vi "Lab Panel V6.00.vi"() -> ()   [LabVIEW 2017] (continued)
                                n860 = local read "SET LAB03-2"() -> (w1506:T5)
                                n861 = case shown="\"T-RISE TEST\"" w1511 {
                                tunnel: ["L03-2-CHART TEST-" "L03-2-CYCLE TEST-" "L03-2-T-RISE TEST-"] -> w1507
                                frame "CHART TEST", Default {
                                }
                                frame "CYCLE TEST" {
                                }
                                frame "T-RISE TEST" {
                                }
                                }
                                n862 = Unbundle(w1506) -> ("DESCRIPTION"=w1505:string)  [unwired: 4 out]
                                n863 = Concatenate Strings(w1501, "\\", w1499, w1497, w1498, w1497) -> (w1508:string)
                                n864 = String To Path(string=w1508) -> (path=w1510:path)
                                n865 = Concatenate Strings(w1508, w1507, w1505, "-", w1504, ".tdms") -> (w1496:string)
                                n866 = Create Folder(path (use dialog)=w1510) -> (error out=w1509:errorcluster)  [unwired: 2 in, 2 out]
                                n867 = global write "Global 1.vi" "LAB03-2 FILE"(w1496) -> ()
                                n868 = call <vilib>:"Clear Errors.vi"("error in (no error)"=w1509) -> ()  [unwired: 5 in, 2 out]
                              }
                              frame #1 {
                                (unwired) FALSE
                                n869 = String To Path(string=w1520) -> (path=w1516:path)
                                n870 = TDMS Open(6:FALSE, 10:T22."create or replace" ("operation (0:open)"), 11:w1516) -> (0:w1515:errorcluster, 3:→"TDMS LAB03-2":refnum<k34>)  [unwired: 4 in]
                              }
                              frame #2 {
                                n871 = local read "SET LAB03-2"() -> (w1526:T5)
                                n872 = local read "TDMS LAB03-2"() -> (w1537:refnum<k34>)
                                n873 = Build Array("Testers Name", "Description", "Set Test Cycles", "T-Rise minutes", "T-Rise Deg C") -> (w1527:string[])
                                n874 = Unbundle(w1526) -> ("NAME"=w1525:string, "DESCRIPTION"=w1524:string, "CYCLES"=w1523:dbl, "T-RISE mins"=w1522:dbl, "T-RISE deg C"=w1521:dbl)
                                n875 = Number To Decimal String(number=w1523) -> (decimal integer string=w1536:string)  [unwired: 1 in]
                                n876 = Number To Decimal String(number=w1522) -> (decimal integer string=w1535:string)  [unwired: 1 in]
                                n877 = Number To Decimal String(number=w1521) -> (decimal integer string=w1534:string)  [unwired: 1 in]
                                n878 = Build Array(w1525, w1524, w1536, w1535, w1534) -> (w1533:string[])
                                n879 = TDMS Set Properties(5:w1533, 7:w1527, 11:w1537) -> ()  [unwired: 3 in, 4 out]
                              }
                              frame #3 {
                                n880 = local read "DISP LAB03-2"() -> (w1542:T4)
                                n881 = Concatenate Strings("LAB03-2  ", w1541) -> (w1543:string)
                                n882 = Two Button Dialog(message=w1543, 1:w1539, 2:w1540) -> (T button?=w1545:bool)
                                n883 = case shown="True" w1545 {
                                tunnel: w1542 -> [w1552 w1553]
                                tunnel: [w1552 w1553] -> w1549
                                tunnel: [w1551 w1554] -> w1548
                                tunnel: [w1550 w1554] -> w1547
                                frame False {
                                n884 = Unbundle(w1552) -> ("CYCLE"=w1551:dbl, "MINS"=w1550:dbl)  [unwired: 1 out]
                                }
                                frame True {
                                w1554 = 0.0
                                }
                                }
                                n885 = Bundle(cluster=w1549, "CYCLE"=w1548, "MINS"=w1547, "STATUS"="RUN") -> (w1538:T4)
                                n886 = local write "DISP LAB03-2"(w1538) -> ()
                              }
                              frame #4 {
                                n887 = local read "TEMP START LAB03-2"() -> (w1557:cluster{"TL":dbl, "TN":dbl})
                                n888 = Bundle(cluster=w1557, "TL"=w1555, "TN"=w1555) -> (w1556:cluster{"TL":dbl, "TN":dbl})
                                n889 = local write "TEMP START LAB03-2"(w1556) -> ()
                              }
                            }
                          }
                        }
                      }
                    }
                  }
                }
              }
              event "RUN LAB04-1": Value Change {
                n890 = event-data() -> ("NewVal"=w1562:bool)  [unwired: 1 in, 5 out]
                n891 = local write "run lab04-1"(w1562) -> ()
                n892 = case shown="True" w1562 {
                  tunnel: w1568 -> [_ w1606]
                  tunnel: w1567 -> [_ w1605]
                  tunnel: w1565 -> [w1570 w1604]
                  tunnel: w1566 -> [_ w1603]
                  tunnel: w1564 -> [_ w1602]
                  tunnel: [w1569 w1601] -> w1563
                  tunnel: w1561 -> [_ w1600]
                  tunnel: w1560 -> [_ w1599]
                  tunnel: w1559 -> [_ w1598]
                  tunnel: w1558 -> [_ w1596]
                  frame False {
                    # "stop test"
                    n893 = stacked-sequence {
                      tunnel: w1570 -> [w1579 _]
                      tunnel: [w1571 _] -> w1569
                      frame #0 {
                        n894 = local read "DISP LAB04-1"() -> (w1578:T4)
                        n895 = Unbundle(w1578) -> ("CYCLE"=w1576:dbl, "MINS"=w1577:dbl)  [unwired: 1 out]
                        n896 = case shown="\"CYCLE TEST\"" w1579 {
                          tunnel: w1577 -> [_ _ w1586]
                          tunnel: w1576 -> [w1584 w1585 _]
                          tunnel: [w1584 w1585 w1586] -> w1575
                          frame "CHART TEST", Default {
                          }
                          frame "CYCLE TEST" {
                          }
                          frame "T-RISE TEST" {
                          }
                        }
                        n897 = local read "TDMS LAB04-1"() -> (w1583:refnum<k34>)
                        n898 = Build Array("STOPPED") -> (w1580:string[])
                        n899 = Build Array(w1575) -> (w1574:dbl[])
                        n900 = TDMS Write(0:w1583, 5:"TEST RESULT", 7:w1580, 9:w1574) -> (4:w1572:refnum<k34>, 15:w1573:errorcluster)  [unwired: 2 in, 2 out]
                        n901 = TDMS Close(8:w1573, 11:w1572) -> (0:w1571:errorcluster)  [unwired: 1 out]
                      }
                      frame #1 {
                        n902 = local read "DISP LAB04-1"() -> (w1590:T4)
                        n903 = stacked-sequence {
                          tunnel: "LAB04-1" -> [w1592 w1594]
                          frame #0 {
                            n904 = call "sub vi - defrag tdms v1.vi"("panel id"=w1592) -> ("error out"=w1591:errorcluster)  [unwired: 10 in]
                            n905 = local write "data file error"(w1591) -> ()
                          }
                          frame #1 {
                            n906 = call "Save data file (stop) v3.vi"("panel id"=w1594) -> ("network file save error"=w1593:errorcluster)  [unwired: 9 in, 1 out]
                            n907 = local write "RESULT LAB04-1"(FALSE) -> ()
                            n908 = local write "data file error"(w1593) -> ()
                          }
                        }
                        n909 = Bundle(cluster=w1590, "STATUS"="STOP") -> (w1588:T4)  [unwired: 2 in]
                        n910 = local write "DISP LAB04-1"(w1588) -> ()
                      }
                    }
                  }
                  frame True {
                    n911 = local read "SIG LAB04-1"() -> (w1597:T2)
                    n912 = stacked-sequence {
                      seq-local: [w1608 _] -> [_ w1612]
                      tunnel: w1606 -> [_ w1622]
                      tunnel: w1605 -> [_ w1621]
                      tunnel: w1604 -> [_ w1620]
                      tunnel: w1603 -> [_ w1619]
                      tunnel: w1602 -> [_ w1618]
                      tunnel: [_ w1617] -> w1601
                      tunnel: w1600 -> [_ w1616]
                      tunnel: w1599 -> [_ w1615]
                      tunnel: w1598 -> [_ w1614]
                      tunnel: w1597 -> [w1607 w1613]
                      tunnel: w1596 -> [_ w1611]
                      frame #0 {
                        n913 = Unbundle(w1607) -> ("AMPS"=w1610:dbl)  [unwired: 4 out]
                        n914 = call "Check For Amps on v1.vi"("ID"="LAB04-1", "amps"=w1610) -> ("amps"=w1608:bool)  [unwired: 9 in]
                      }
                      frame #1 {
                        n915 = case shown="True" w1612 {
                          tunnel: w1622 -> [_ w1635]
                          tunnel: w1621 -> [_ w1634]
                          tunnel: w1620 -> [_ w1633]
                          tunnel: w1619 -> [_ w1632]
                          tunnel: w1618 -> [_ w1631]
                          tunnel: [errorcluster {"status"=FALSE, "code"=0, "source"=""} ("error out") w1630] -> w1617
                          tunnel: w1616 -> [_ w1629]
                          tunnel: w1615 -> [_ w1628]
                          tunnel: w1614 -> [_ w1627]
                          tunnel: w1613 -> [_ w1626]
                          tunnel: w1611 -> [_ w1625]
                          frame False {
                            w1623 = FALSE
                            n916 = local write "RUN LAB04-1"(w1623) -> ()
                            n917 = local write "run lab04-1"(w1623) -> ()
                          }
                          frame True {
                            n918 = stacked-sequence {
                              seq-local: [w1636 _ _ _ _] -> [_ w1660 _ _ _]
                              tunnel: w1635 -> [w1641 _ _ _ _]
                              tunnel: w1634 -> [w1637 _ _ _ _]
                              tunnel: w1633 -> [w1651 _ _ _ _]
                              tunnel: w1632 -> [w1644 _ _ _ _]
                              tunnel: w1631 -> [w1639 _ _ _ _]
                              tunnel: [_ w1655 _ _ _] -> w1630
                              tunnel: w1629 -> [_ _ _ w1681 _]
                              tunnel: w1628 -> [_ _ _ w1680 _]
                              tunnel: w1627 -> [_ _ _ w1679 _]
                              tunnel: w1626 -> [_ _ _ _ _]
                              tunnel: w1625 -> [_ _ _ _ w1695]
                              frame #0 {
                                w1638 = "\\"
                                n919 = local read "SET LAB04-1"() -> (w1646:T5)
                                n920 = case shown="\"CYCLE TEST\"" w1651 {
                                tunnel: ["L04-1-CHART TEST-" "L04-1-CYCLE TEST-" "L04-1-T-RISE TEST-"] -> w1647
                                frame "CHART TEST", Default {
                                }
                                frame "CYCLE TEST" {
                                }
                                frame "T-RISE TEST" {
                                }
                                }
                                n921 = Unbundle(w1646) -> ("DESCRIPTION"=w1645:string)  [unwired: 4 out]
                                n922 = Concatenate Strings(w1641, "\\", w1639, w1638, w1637, w1638) -> (w1648:string)
                                n923 = String To Path(string=w1648) -> (path=w1650:path)
                                n924 = Concatenate Strings(w1648, w1647, w1645, "-", w1644, ".tdms") -> (w1636:string)
                                n925 = Create Folder(path (use dialog)=w1650) -> (error out=w1649:errorcluster)  [unwired: 2 in, 2 out]
                                n926 = global write "Global 1.vi" "LAB04-1 FILE"(w1636) -> ()
                                n927 = call <vilib>:"Clear Errors.vi"("error in (no error)"=w1649) -> ()  [unwired: 5 in, 2 out]
                              }
                              frame #1 {
                                (unwired) FALSE
                                n928 = String To Path(string=w1660) -> (path=w1656:path)
                                n929 = TDMS Open(6:FALSE, 10:T22."create or replace" ("operation (0:open)"), 11:w1656) -> (0:w1655:errorcluster, 3:→"TDMS LAB04-1":refnum<k34>)  [unwired: 4 in]
                              }
                              frame #2 {
                                n930 = local read "SET LAB04-1"() -> (w1666:T5)
                                n931 = local read "TDMS LAB04-1"() -> (w1677:refnum<k34>)
                                n932 = Build Array("Testers Name", "Description", "Set Test Cycles", "T-Rise minutes", "T-Rise Deg C") -> (w1667:string[])
                                n933 = Unbundle(w1666) -> ("NAME"=w1665:string, "DESCRIPTION"=w1664:string, "CYCLES"=w1663:dbl, "T-RISE mins"=w1662:dbl, "T-RISE deg C"=w1661:dbl)
                                n934 = Number To Decimal String(number=w1663) -> (decimal integer string=w1676:string)  [unwired: 1 in]
                                n935 = Number To Decimal String(number=w1662) -> (decimal integer string=w1675:string)  [unwired: 1 in]
                                n936 = Number To Decimal String(number=w1661) -> (decimal integer string=w1674:string)  [unwired: 1 in]
                                n937 = Build Array(w1665, w1664, w1676, w1675, w1674) -> (w1673:string[])
                                n938 = TDMS Set Properties(5:w1673, 7:w1667, 11:w1677) -> ()  [unwired: 3 in, 4 out]
                              }
                              frame #3 {
                                n939 = local read "DISP LAB04-1"() -> (w1682:T4)
                                n940 = Concatenate Strings("LAB04-1  ", w1681) -> (w1683:string)
                                n941 = Two Button Dialog(message=w1683, 1:w1679, 2:w1680) -> (T button?=w1685:bool)
                                n942 = case shown="True" w1685 {
                                tunnel: w1682 -> [w1692 w1693]
                                tunnel: [w1692 w1693] -> w1689
                                tunnel: [w1691 w1694] -> w1688
                                tunnel: [w1690 w1694] -> w1687
                                frame False {
                                n943 = Unbundle(w1692) -> ("CYCLE"=w1691:dbl, "MINS"=w1690:dbl)  [unwired: 1 out]
                                }
                                frame True {
                                w1694 = 0.0
                                }
                                }
                                n944 = Bundle(cluster=w1689, "CYCLE"=w1688, "MINS"=w1687, "STATUS"="RUN") -> (w1678:T4)
                                n945 = local write "DISP LAB04-1"(w1678) -> ()
                              }
                              frame #4 {
                                n946 = local read "TEMP START LAB04-1"() -> (w1697:cluster{"TL":dbl, "TN":dbl})
                                n947 = Bundle(cluster=w1697, "TL"=w1695, "TN"=w1695) -> (w1696:cluster{"TL":dbl, "TN":dbl})
                                n948 = local write "TEMP START LAB04-1"(w1696) -> ()
                              }
                            }
                          }
                        }
                      }
                    }
                  }
                }
              }
              event "RUN LAB04-2": Value Change {
                n949 = event-data() -> ("NewVal"=w1702:bool)  [unwired: 1 in, 5 out]
                n950 = local write "run lab04-2"(w1702) -> ()
                n951 = case shown="True" w1702 {
                  tunnel: w1708 -> [_ w1746]
                  tunnel: w1707 -> [_ w1745]
                  tunnel: w1705 -> [w1710 w1744]
                  tunnel: w1706 -> [_ w1743]
                  tunnel: w1704 -> [_ w1742]
                  tunnel: [w1709 w1741] -> w1703
                  tunnel: w1701 -> [_ w1740]
                  tunnel: w1700 -> [_ w1739]
                  tunnel: w1699 -> [_ w1738]
                  tunnel: w1698 -> [_ w1736]
                  frame False {
                    # "stop test"
                    n952 = stacked-sequence {
                      tunnel: w1710 -> [w1719 _]
                      tunnel: [w1711 _] -> w1709
                      frame #0 {
                        n953 = local read "DISP LAB04-2"() -> (w1718:T4)
                        n954 = Unbundle(w1718) -> ("CYCLE"=w1716:dbl, "MINS"=w1717:dbl)  [unwired: 1 out]
                        n955 = case shown="\"CYCLE TEST\"" w1719 {
                          tunnel: w1717 -> [_ _ w1726]
                          tunnel: w1716 -> [w1724 w1725 _]
                          tunnel: [w1724 w1725 w1726] -> w1715
                          frame "CHART TEST", Default {
                          }
                          frame "CYCLE TEST" {
                          }
                          frame "T-RISE TEST" {
                          }
                        }
                        n956 = local read "TDMS LAB04-2"() -> (w1723:refnum<k34>)
                        n957 = Build Array("STOPPED") -> (w1720:string[])
                        n958 = Build Array(w1715) -> (w1714:dbl[])
                        n959 = TDMS Write(0:w1723, 5:"TEST RESULT", 7:w1720, 9:w1714) -> (4:w1712:refnum<k34>, 15:w1713:errorcluster)  [unwired: 2 in, 2 out]
                        n960 = TDMS Close(8:w1713, 11:w1712) -> (0:w1711:errorcluster)  [unwired: 1 out]
                      }
                      frame #1 {
                        n961 = local read "DISP LAB04-2"() -> (w1730:T4)
                        n962 = stacked-sequence {
                          tunnel: "LAB04-2" -> [w1732 w1734]
                          frame #0 {
                            n963 = call "sub vi - defrag tdms v1.vi"("panel id"=w1732) -> ("error out"=w1731:errorcluster)  [unwired: 10 in]
                            n964 = local write "data file error"(w1731) -> ()
                          }
                          frame #1 {
                            n965 = call "Save data file (stop) v3.vi"("panel id"=w1734) -> ("network file save error"=w1733:errorcluster)  [unwired: 9 in, 1 out]
                            n966 = local write "RESULT LAB04-2"(FALSE) -> ()
                            n967 = local write "data file error"(w1733) -> ()
                          }
                        }
                        n968 = Bundle(cluster=w1730, "STATUS"="STOP") -> (w1728:T4)  [unwired: 2 in]
                        n969 = local write "DISP LAB04-2"(w1728) -> ()
                      }
                    }
                  }
                  frame True {
                    n970 = local read "SIG LAB04-2"() -> (w1737:T2)
                    n971 = stacked-sequence {
                      seq-local: [w1748 _] -> [_ w1752]
                      tunnel: w1746 -> [_ w1762]
                      tunnel: w1745 -> [_ w1761]
                      tunnel: w1744 -> [_ w1760]
                      tunnel: w1743 -> [_ w1759]
                      tunnel: w1742 -> [_ w1758]
                      tunnel: [_ w1757] -> w1741
                      tunnel: w1740 -> [_ w1756]
                      tunnel: w1739 -> [_ w1755]
                      tunnel: w1738 -> [_ w1754]
                      tunnel: w1737 -> [w1747 w1753]
                      tunnel: w1736 -> [_ w1751]
                      frame #0 {
                        n972 = Unbundle(w1747) -> ("AMPS"=w1750:dbl)  [unwired: 4 out]
                        n973 = call "Check For Amps on v1.vi"("ID"="LAB04-2", "amps"=w1750) -> ("amps"=w1748:bool)  [unwired: 9 in]
                      }
                      frame #1 {
                        n974 = case shown="True" w1752 {
                          tunnel: w1762 -> [_ w1775]
                          tunnel: w1761 -> [_ w1774]
                          tunnel: w1760 -> [_ w1773]
                          tunnel: w1759 -> [_ w1772]
                          tunnel: w1758 -> [_ w1771]
                          tunnel: [errorcluster {"status"=FALSE, "code"=0, "source"=""} ("error out") w1770] -> w1757
                          tunnel: w1756 -> [_ w1769]
                          tunnel: w1755 -> [_ w1768]
                          tunnel: w1754 -> [_ w1767]
                          tunnel: w1753 -> [_ w1766]
                          tunnel: w1751 -> [_ w1765]
                          frame False {
                            w1763 = FALSE
                            n975 = local write "RUN LAB04-2"(w1763) -> ()
                            n976 = local write "run lab04-2"(w1763) -> ()
                          }
                          frame True {
                            n977 = stacked-sequence {
                              seq-local: [w1776 _ _ _ _] -> [_ w1800 _ _ _]
                              tunnel: w1775 -> [w1781 _ _ _ _]
                              tunnel: w1774 -> [w1777 _ _ _ _]
                              tunnel: w1773 -> [w1791 _ _ _ _]
                              tunnel: w1772 -> [w1784 _ _ _ _]
                              tunnel: w1771 -> [w1779 _ _ _ _]
                              tunnel: [_ w1795 _ _ _] -> w1770
                              tunnel: w1769 -> [_ _ _ w1821 _]
                              tunnel: w1768 -> [_ _ _ w1820 _]
                              tunnel: w1767 -> [_ _ _ w1819 _]
                              tunnel: w1766 -> [_ _ _ _ _]
                              tunnel: w1765 -> [_ _ _ _ w1835]
                              frame #0 {
                                w1778 = "\\"
                                n978 = local read "SET LAB04-2"() -> (w1786:T5)
                                n979 = case shown="\"CHART TEST\", Default" w1791 {
                                tunnel: ["L04-2-CHART TEST-" "L04-2-CYCLE TEST-" "L04-2-T-RISE TEST-"] -> w1787
                                frame "CHART TEST", Default {
                                }
                                frame "CYCLE TEST" {
                                }
                                frame "T-RISE TEST" {
                                }
                                }
                                n980 = Unbundle(w1786) -> ("DESCRIPTION"=w1785:string)  [unwired: 4 out]
                                n981 = Concatenate Strings(w1781, "\\", w1779, w1778, w1777, w1778) -> (w1788:string)
                                n982 = String To Path(string=w1788) -> (path=w1790:path)
                                n983 = Concatenate Strings(w1788, w1787, w1785, "-", w1784, ".tdms") -> (w1776:string)
                                n984 = Create Folder(path (use dialog)=w1790) -> (error out=w1789:errorcluster)  [unwired: 2 in, 2 out]
                                n985 = global write "Global 1.vi" "LAB04-2 FILE"(w1776) -> ()
                                n986 = call <vilib>:"Clear Errors.vi"("error in (no error)"=w1789) -> ()  [unwired: 5 in, 2 out]
                              }
                              frame #1 {
                                (unwired) FALSE
                                n987 = String To Path(string=w1800) -> (path=w1796:path)
                                n988 = TDMS Open(6:FALSE, 10:T22."create or replace" ("operation (0:open)"), 11:w1796) -> (0:w1795:errorcluster, 3:→"TDMS LAB04-2":refnum<k34>)  [unwired: 4 in]
                              }
                              frame #2 {
                                n989 = local read "SET LAB04-2"() -> (w1806:T5)
                                n990 = local read "TDMS LAB04-2"() -> (w1817:refnum<k34>)
                                n991 = Build Array("Testers Name", "Description", "Set Test Cycles", "T-Rise minutes", "T-Rise Deg C") -> (w1807:string[])
                                n992 = Unbundle(w1806) -> ("NAME"=w1805:string, "DESCRIPTION"=w1804:string, "CYCLES"=w1803:dbl, "T-RISE mins"=w1802:dbl, "T-RISE deg C"=w1801:dbl)
                                n993 = Number To Decimal String(number=w1803) -> (decimal integer string=w1816:string)  [unwired: 1 in]
                                n994 = Number To Decimal String(number=w1802) -> (decimal integer string=w1815:string)  [unwired: 1 in]
                                n995 = Number To Decimal String(number=w1801) -> (decimal integer string=w1814:string)  [unwired: 1 in]
                                n996 = Build Array(w1805, w1804, w1816, w1815, w1814) -> (w1813:string[])
                                n997 = TDMS Set Properties(5:w1813, 7:w1807, 11:w1817) -> ()  [unwired: 3 in, 4 out]
                              }
                              frame #3 {
                                n998 = local read "DISP LAB04-2"() -> (w1822:T4)
                                n999 = Concatenate Strings("LAB04-2 ", w1821) -> (w1823:string)
                                n1000 = Two Button Dialog(message=w1823, 1:w1819, 2:w1820) -> (T button?=w1825:bool)
                                n1001 = case shown="True" w1825 {
                                tunnel: w1822 -> [w1832 w1833]
                                tunnel: [w1832 w1833] -> w1829
                                tunnel: [w1831 w1834] -> w1828
                                tunnel: [w1830 w1834] -> w1827
                                frame False {
                                n1002 = Unbundle(w1832) -> ("CYCLE"=w1831:dbl, "MINS"=w1830:dbl)  [unwired: 1 out]
                                }
                                frame True {
                                w1834 = 0.0
                                }
                                }
                                n1003 = Bundle(cluster=w1829, "CYCLE"=w1828, "MINS"=w1827, "STATUS"="RUN") -> (w1818:T4)
                                n1004 = local write "DISP LAB04-2"(w1818) -> ()
                              }
                              frame #4 {
                                n1005 = local read "TEMP START LAB04-2"() -> (w1837:cluster{"TL":dbl, "TN":dbl})
                                n1006 = Bundle(cluster=w1837, "TL"=w1835, "TN"=w1835) -> (w1836:cluster{"TL":dbl, "TN":dbl})
                                n1007 = local write "TEMP START LAB04-2"(w1836) -> ()
                              }
                            }
                          }
                        }
                      }
                    }
                  }
                }
              }
              event "RUN LAB05-1": Value Change {
                n1008 = event-data() -> ("NewVal"=w1842:bool)  [unwired: 1 in, 5 out]
                n1009 = local write "run lab05-1"(w1842) -> ()
                n1010 = case shown="True" w1842 {
                  tunnel: w1848 -> [_ w1886]
                  tunnel: w1847 -> [_ w1885]
                  tunnel: w1845 -> [w1850 w1884]
                  tunnel: w1846 -> [_ w1883]
                  tunnel: w1844 -> [_ w1882]
                  tunnel: [w1849 w1881] -> w1843
                  tunnel: w1841 -> [_ w1880]
                  tunnel: w1840 -> [_ w1879]
                  tunnel: w1839 -> [_ w1878]
                  tunnel: w1838 -> [_ w1876]
                  frame False {
                    # "stop test"
                    n1011 = stacked-sequence {
                      tunnel: w1850 -> [w1859 _]
                      tunnel: [w1851 _] -> w1849
                      frame #0 {
                        n1012 = local read "DISP LAB05-1"() -> (w1858:T4)
                        n1013 = Unbundle(w1858) -> ("CYCLE"=w1856:dbl, "MINS"=w1857:dbl)  [unwired: 1 out]
                        n1014 = case shown="\"CYCLE TEST\"" w1859 {
                          tunnel: w1857 -> [_ _ w1866]
                          tunnel: w1856 -> [w1864 w1865 _]
                          tunnel: [w1864 w1865 w1866] -> w1855
                          frame "CHART TEST", Default {
                          }
                          frame "CYCLE TEST" {
                          }
                          frame "T-RISE TEST" {
                          }
                        }
                        n1015 = local read "TDMS LAB05-1"() -> (w1863:refnum<k34>)
                        n1016 = Build Array("STOPPED") -> (w1860:string[])
                        n1017 = Build Array(w1855) -> (w1854:dbl[])
                        n1018 = TDMS Write(0:w1863, 5:"TEST RESULT", 7:w1860, 9:w1854) -> (4:w1852:refnum<k34>, 15:w1853:errorcluster)  [unwired: 2 in, 2 out]
                        n1019 = TDMS Close(8:w1853, 11:w1852) -> (0:w1851:errorcluster)  [unwired: 1 out]
                      }
                      frame #1 {
                        n1020 = local read "DISP LAB05-1"() -> (w1870:T4)
                        n1021 = stacked-sequence {
                          tunnel: "LAB05-1" -> [w1872 w1874]
                          frame #0 {
                            n1022 = call "sub vi - defrag tdms v1.vi"("panel id"=w1872) -> ("error out"=w1871:errorcluster)  [unwired: 10 in]
                            n1023 = local write "data file error"(w1871) -> ()
                          }
                          frame #1 {
                            n1024 = call "Save data file (stop) v3.vi"("panel id"=w1874) -> ("network file save error"=w1873:errorcluster)  [unwired: 9 in, 1 out]
                            n1025 = local write "RESULT LAB05-1"(FALSE) -> ()
                            n1026 = local write "data file error"(w1873) -> ()
                          }
                        }
                        n1027 = Bundle(cluster=w1870, "STATUS"="STOP") -> (w1868:T4)  [unwired: 2 in]
                        n1028 = local write "DISP LAB05-1"(w1868) -> ()
                      }
                    }
                  }
                  frame True {
                    n1029 = local read "SIG LAB05-1"() -> (w1877:T2)
                    n1030 = stacked-sequence {
                      seq-local: [w1888 _] -> [_ w1892]
                      tunnel: w1886 -> [_ w1902]
                      tunnel: w1885 -> [_ w1901]
                      tunnel: w1884 -> [_ w1900]
                      tunnel: w1883 -> [_ w1899]
                      tunnel: w1882 -> [_ w1898]
                      tunnel: [_ w1897] -> w1881
                      tunnel: w1880 -> [_ w1896]
                      tunnel: w1879 -> [_ w1895]
                      tunnel: w1878 -> [_ w1894]
                      tunnel: w1877 -> [w1887 w1893]
                      tunnel: w1876 -> [_ w1891]
                      frame #0 {
                        n1031 = Unbundle(w1887) -> ("AMPS"=w1890:dbl)  [unwired: 4 out]
                        n1032 = call "Check For Amps on v1.vi"("ID"="LAB05-1", "amps"=w1890) -> ("amps"=w1888:bool)  [unwired: 9 in]
                      }
                      frame #1 {
                        n1033 = case shown="True" w1892 {
                          tunnel: w1902 -> [_ w1915]
                          tunnel: w1901 -> [_ w1914]
                          tunnel: w1900 -> [_ w1913]
                          tunnel: w1899 -> [_ w1912]
                          tunnel: w1898 -> [_ w1911]
                          tunnel: [errorcluster {"status"=FALSE, "code"=0, "source"=""} ("error out") w1910] -> w1897
                          tunnel: w1896 -> [_ w1909]
                          tunnel: w1895 -> [_ w1908]
                          tunnel: w1894 -> [_ w1907]
                          tunnel: w1893 -> [_ w1906]
                          tunnel: w1891 -> [_ w1905]
                          frame False {
                            w1903 = FALSE
                            n1034 = local write "RUN LAB05-1"(w1903) -> ()
                            n1035 = local write "run lab05-1"(w1903) -> ()
                          }
                          frame True {
                            n1036 = stacked-sequence {
                              seq-local: [w1916 _ _ _ _] -> [_ w1940 _ _ _]
                              tunnel: w1915 -> [w1921 _ _ _ _]
                              tunnel: w1914 -> [w1917 _ _ _ _]
                              tunnel: w1913 -> [w1931 _ _ _ _]
                              tunnel: w1912 -> [w1924 _ _ _ _]
                              tunnel: w1911 -> [w1919 _ _ _ _]
                              tunnel: [_ w1935 _ _ _] -> w1910
                              tunnel: w1909 -> [_ _ _ w1960 _]
                              tunnel: w1908 -> [_ _ _ w1959 _]
                              tunnel: w1907 -> [_ _ _ w1958 _]
                              tunnel: w1906 -> [_ _ _ _ _]
                              tunnel: w1905 -> [_ _ _ _ w1975]
                              frame #0 {
                                w1918 = "\\"
                                n1037 = local read "SET LAB05-1"() -> (w1926:T5)
                                n1038 = case shown="\"CYCLE TEST\"" w1931 {
                                tunnel: ["L05-1-CHART TEST-" "L05-1-CYCLE TEST-" "L05-1-T-RISE TEST-"] -> w1927
                                frame "CHART TEST", Default {
                                }
                                frame "CYCLE TEST" {
                                }
                                frame "T-RISE TEST" {
                                }
                                }
                                n1039 = Unbundle(w1926) -> ("DESCRIPTION"=w1925:string)  [unwired: 4 out]
                                n1040 = Concatenate Strings(w1921, "\\", w1919, w1918, w1917, w1918) -> (w1928:string)
                                n1041 = String To Path(string=w1928) -> (path=w1930:path)
                                n1042 = Concatenate Strings(w1928, w1927, w1925, "-", w1924, ".tdms") -> (w1916:string)
                                n1043 = Create Folder(path (use dialog)=w1930) -> (error out=w1929:errorcluster)  [unwired: 2 in, 2 out]
                                n1044 = global write "Global 1.vi" "LAB05-1 FILE"(w1916) -> ()
                                n1045 = call <vilib>:"Clear Errors.vi"("error in (no error)"=w1929) -> ()  [unwired: 5 in, 2 out]
                              }
                              frame #1 {
                                (unwired) FALSE
                                n1046 = String To Path(string=w1940) -> (path=w1936:path)
                                n1047 = TDMS Open(6:FALSE, 10:T22."create or replace" ("operation (0:open)"), 11:w1936) -> (0:w1935:errorcluster, 3:→"TDMS LAB05-1":refnum<k34>)  [unwired: 4 in]
                              }
                              frame #2 {
                                n1048 = local read "SET LAB05-1"() -> (w1946:T5)
                                n1049 = local read "TDMS LAB05-1"() -> (w1957:refnum<k34>)
                                n1050 = Build Array("Testers Name", "Description", "Set Test Cycles", "T-Rise minutes", "T-Rise Deg C") -> (w1947:string[])
                                n1051 = Unbundle(w1946) -> ("NAME"=w1945:string, "DESCRIPTION"=w1944:string, "CYCLES"=w1943:dbl, "T-RISE mins"=w1942:dbl, "T-RISE deg C"=w1941:dbl)
                                n1052 = Number To Decimal String(number=w1943) -> (decimal integer string=w1956:string)  [unwired: 1 in]
                                n1053 = Number To Decimal String(number=w1942) -> (decimal integer string=w1955:string)  [unwired: 1 in]
                                n1054 = Number To Decimal String(number=w1941) -> (decimal integer string=w1954:string)  [unwired: 1 in]
                                n1055 = Build Array(w1945, w1944, w1956, w1955, w1954) -> (w1953:string[])
                                n1056 = TDMS Set Properties(5:w1953, 7:w1947, 11:w1957) -> ()  [unwired: 3 in, 4 out]
                              }
                              frame #3 {
                                n1057 = local read "DISP LAB05-1"() -> (w1962:T4)
                                n1058 = Concatenate Strings("LAB05-1  ", w1960) -> (w1963:string)
                                n1059 = Two Button Dialog(message=w1963, 1:w1958, 2:w1959) -> (T button?=w1965:bool)
                                n1060 = case shown="True" w1965 {
                                tunnel: w1962 -> [w1972 w1973]
                                tunnel: [w1972 w1973] -> w1969
                                tunnel: [w1971 w1974] -> w1968
                                tunnel: [w1970 w1974] -> w1967
                                frame False {
                                n1061 = Unbundle(w1972) -> ("CYCLE"=w1971:dbl, "MINS"=w1970:dbl)  [unwired: 1 out]
                                }
                                frame True {
                                w1974 = 0.0
                                }
                                }
                                n1062 = Bundle(cluster=w1969, "CYCLE"=w1968, "MINS"=w1967, "STATUS"="RUN") -> (w1961:T4)
                                n1063 = local write "DISP LAB05-1"(w1961) -> ()
                              }
                              frame #4 {
                                n1064 = local read "TEMP START LAB05-1"() -> (w1977:cluster{"TL":dbl, "TN":dbl})
                                n1065 = Bundle(cluster=w1977, "TL"=w1975, "TN"=w1975) -> (w1976:cluster{"TL":dbl, "TN":dbl})
                                n1066 = local write "TEMP START LAB05-1"(w1976) -> ()
                              }
                            }
                          }
                        }
                      }
                    }
                  }
                }
              }
              event "RUN LAB05-2": Value Change {
                n1067 = event-data() -> ("NewVal"=w1983:bool)  [unwired: 1 in, 5 out]
                n1068 = local read "SIG LAB05-2"() -> (w1979:T2)
                n1069 = case shown="True" w1983 {
                  tunnel: w1989 -> [_ w2027]
                  tunnel: w1988 -> [_ w2026]
                  tunnel: w1986 -> [w1991 w2025]
                  tunnel: w1987 -> [_ w2024]
                  tunnel: w1985 -> [_ w2023]
                  tunnel: [w1990 w2022] -> w1984
                  tunnel: w1982 -> [_ w2021]
                  tunnel: w1981 -> [_ w2020]
                  tunnel: w1980 -> [_ w2019]
                  tunnel: w1979 -> [_ w2018]
                  tunnel: w1978 -> [_ w2017]
                  frame False {
                    # "stop test"
                    n1070 = stacked-sequence {
                      tunnel: w1991 -> [w2000 _]
                      tunnel: [w1992 _] -> w1990
                      frame #0 {
                        n1071 = local read "DISP LAB05-2"() -> (w1999:T4)
                        n1072 = Unbundle(w1999) -> ("CYCLE"=w1997:dbl, "MINS"=w1998:dbl)  [unwired: 1 out]
                        n1073 = case shown="\"CYCLE TEST\"" w2000 {
                          tunnel: w1998 -> [_ _ w2007]
                          tunnel: w1997 -> [w2005 w2006 _]
                          tunnel: [w2005 w2006 w2007] -> w1996
                          frame "CHART TEST", Default {
                          }
                          frame "CYCLE TEST" {
                          }
                          frame "T-RISE TEST" {
                          }
                        }
                        n1074 = local read "TDMS LAB05-2"() -> (w2004:refnum<k34>)
                        n1075 = Build Array("STOPPED") -> (w2001:string[])
                        n1076 = Build Array(w1996) -> (w1995:dbl[])
                        n1077 = TDMS Write(0:w2004, 5:"TEST RESULT", 7:w2001, 9:w1995) -> (4:w1993:refnum<k34>, 15:w1994:errorcluster)  [unwired: 2 in, 2 out]
                        n1078 = TDMS Close(8:w1994, 11:w1993) -> (0:w1992:errorcluster)  [unwired: 1 out]
                      }
                      frame #1 {
                        n1079 = local read "DISP LAB05-2"() -> (w2011:T4)
                        n1080 = stacked-sequence {
                          tunnel: "LAB05-2" -> [w2013 w2015]
                          frame #0 {
                            n1081 = call "sub vi - defrag tdms v1.vi"("panel id"=w2013) -> ("error out"=w2012:errorcluster)  [unwired: 10 in]
                            n1082 = local write "data file error"(w2012) -> ()
                          }
                          frame #1 {
                            n1083 = local write "RESULT LAB05-2"(FALSE) -> ()
                            n1084 = call "Save data file (stop) v3.vi"("panel id"=w2015) -> ("network file save error"=w2014:errorcluster)  [unwired: 9 in, 1 out]
                            n1085 = local write "data file error"(w2014) -> ()
                          }
                        }
                        n1086 = Bundle(cluster=w2011, "STATUS"="STOP") -> (w2009:T4)  [unwired: 2 in]
                        n1087 = local write "DISP LAB05-2"(w2009) -> ()
                      }
                    }
                  }
                  frame True {
                    n1088 = stacked-sequence {
                      seq-local: [w2029 _] -> [_ w2033]
                      tunnel: w2027 -> [_ w2043]
                      tunnel: w2026 -> [_ w2042]
                      tunnel: w2025 -> [_ w2041]
                      tunnel: w2024 -> [_ w2040]
                      tunnel: w2023 -> [_ w2039]
                      tunnel: [_ w2038] -> w2022
                      tunnel: w2021 -> [_ w2037]
                      tunnel: w2020 -> [_ w2036]
                      tunnel: w2019 -> [_ w2035]
                      tunnel: w2018 -> [w2028 w2034]
                      tunnel: w2017 -> [_ w2032]
                      frame #0 {
                        n1089 = Unbundle(w2028) -> ("AMPS"=w2031:dbl)  [unwired: 4 out]
                        n1090 = call "Check For Amps on v1.vi"("ID"="LAB05-2", "amps"=w2031) -> ("amps"=w2029:bool)  [unwired: 9 in]
                      }
                      frame #1 {
                        n1091 = case shown="True" w2033 {
                          tunnel: w2043 -> [_ w2055]
                          tunnel: w2042 -> [_ w2053]
                          tunnel: w2041 -> [_ w2050]
                          tunnel: w2040 -> [_ w2051]
                          tunnel: w2039 -> [_ w2054]
                          tunnel: [errorcluster {"status"=FALSE, "code"=0, "source"=""} ("error out") w2046] -> w2038
                          tunnel: w2037 -> [_ w2049]
                          tunnel: w2036 -> [_ w2048]
                          tunnel: w2035 -> [_ w2047]
                          tunnel: w2034 -> [_ w2052]
                          tunnel: w2032 -> [_ w2056]
                          frame False {
                            w2044 = FALSE
                            n1092 = local write "RUN LAB05-2"(w2044) -> ()
                            n1093 = local write "run lab05-2"(w2044) -> ()
                          }
                          frame True {
                            n1094 = stacked-sequence {
                              seq-local: [w2057 _ _ _ _] -> [_ w2081 _ _ _]
                              tunnel: w2055 -> [w2062 _ _ _ _]
                              tunnel: w2053 -> [w2058 _ _ _ _]
                              tunnel: w2050 -> [w2072 _ _ _ _]
                              tunnel: w2051 -> [w2065 _ _ _ _]
                              tunnel: w2054 -> [w2060 _ _ _ _]
                              tunnel: [_ w2076 _ _ _] -> w2046
                              tunnel: w2049 -> [_ _ _ w2101 _]
                              tunnel: w2048 -> [_ _ _ w2100 _]
                              tunnel: w2047 -> [_ _ _ w2099 _]
                              tunnel: w2052 -> [_ _ _ _ _]
                              tunnel: w2056 -> [_ _ _ _ w2116]
                              frame #0 {
                                w2059 = "\\"
                                n1095 = local read "SET LAB05-2"() -> (w2067:T5)
                                n1096 = case shown="\"CYCLE TEST\"" w2072 {
                                tunnel: ["L05-2-CHART TEST-" "L05-2-CYCLE TEST-" "L05-2-T-RISE TEST-"] -> w2068
                                frame "CHART TEST", Default {
                                }
                                frame "CYCLE TEST" {
                                }
                                frame "T-RISE TEST" {
                                }
                                }
                                n1097 = Unbundle(w2067) -> ("DESCRIPTION"=w2066:string)  [unwired: 4 out]
                                n1098 = Concatenate Strings(w2062, "\\", w2060, w2059, w2058, w2059) -> (w2069:string)
                                n1099 = String To Path(string=w2069) -> (path=w2071:path)
                                n1100 = Concatenate Strings(w2069, w2068, w2066, "-", w2065, ".tdms") -> (w2057:string)
                                n1101 = Create Folder(path (use dialog)=w2071) -> (error out=w2070:errorcluster)  [unwired: 2 in, 2 out]
                                n1102 = global write "Global 1.vi" "LAB05-2 FILE"(w2057) -> ()
                                n1103 = call <vilib>:"Clear Errors.vi"("error in (no error)"=w2070) -> ()  [unwired: 5 in, 2 out]
                              }
                              frame #1 {
                                (unwired) FALSE
                                n1104 = String To Path(string=w2081) -> (path=w2077:path)
                                n1105 = TDMS Open(6:FALSE, 10:T22."create or replace" ("operation (0:open)"), 11:w2077) -> (0:w2076:errorcluster, 3:→"TDMS LAB05-2":refnum<k34>)  [unwired: 4 in]
                              }
                              frame #2 {
                                n1106 = local read "SET LAB05-2"() -> (w2087:T5)
                                n1107 = local read "TDMS LAB05-2"() -> (w2098:refnum<k34>)
                                n1108 = Build Array("Testers Name", "Description", "Set Test Cycles", "T-Rise minutes", "T-Rise Deg C") -> (w2088:string[])
                                n1109 = Unbundle(w2087) -> ("NAME"=w2086:string, "DESCRIPTION"=w2085:string, "CYCLES"=w2084:dbl, "T-RISE mins"=w2083:dbl, "T-RISE deg C"=w2082:dbl)
                                n1110 = Number To Decimal String(number=w2084) -> (decimal integer string=w2097:string)  [unwired: 1 in]
                                n1111 = Number To Decimal String(number=w2083) -> (decimal integer string=w2096:string)  [unwired: 1 in]
                                n1112 = Number To Decimal String(number=w2082) -> (decimal integer string=w2095:string)  [unwired: 1 in]
                                n1113 = Build Array(w2086, w2085, w2097, w2096, w2095) -> (w2094:string[])
                                n1114 = TDMS Set Properties(5:w2094, 7:w2088, 11:w2098) -> ()  [unwired: 3 in, 4 out]
                              }
                              frame #3 {
                                n1115 = local read "DISP LAB05-2"() -> (w2103:T4)
                                n1116 = Concatenate Strings("LAB05-2  ", w2101) -> (w2104:string)
                                n1117 = Two Button Dialog(message=w2104, 1:w2099, 2:w2100) -> (T button?=w2106:bool)
                                n1118 = case shown="True" w2106 {
                                tunnel: w2103 -> [w2113 w2114]
                                tunnel: [w2113 w2114] -> w2110
                                tunnel: [w2112 w2115] -> w2109
                                tunnel: [w2111 w2115] -> w2108
                                frame False {
                                n1119 = Unbundle(w2113) -> ("CYCLE"=w2112:dbl, "MINS"=w2111:dbl)  [unwired: 1 out]
                                }
                                frame True {
                                w2115 = 0.0
                                }
                                }
                                n1120 = Bundle(cluster=w2110, "CYCLE"=w2109, "MINS"=w2108, "STATUS"="RUN") -> (w2102:T4)
                                n1121 = local write "DISP LAB05-2"(w2102) -> ()
                              }
                              frame #4 {
                                n1122 = local read "TEMP START LAB05-2"() -> (w2118:cluster{"TL":dbl, "TN":dbl})
                                n1123 = Bundle(cluster=w2118, "TL"=w2116, "TN"=w2116) -> (w2117:cluster{"TL":dbl, "TN":dbl})
                                n1124 = local write "TEMP START LAB05-2"(w2117) -> ()
                              }
                            }
                          }
                        }
                      }
                    }
                  }
                }
                n1125 = local write "run lab05-2"(w1983) -> ()
              }
            }
            n1126 = local write "data file error"(w687) -> ()
          }
          frame #5 {
            # "Check if test cycles reached for cycle tests, if so then test pass"
            n1127 = stacked-sequence {
              tunnel: w2138 -> [_ _ _ _ _ _ _ _ _ _]
              tunnel: w2137 -> [_ _ _ _ _ _ _ _ _ _]
              tunnel: w2136 -> [_ _ _ _ _ _ _ _ _ _]
              tunnel: w2135 -> [_ _ _ _ _ _ _ _ _ _]
              tunnel: w2134 -> [_ _ _ _ _ _ _ _ _ _]
              tunnel: w2133 -> [_ _ _ _ _ _ _ _ _ _]
              tunnel: w2132 -> [_ _ _ _ _ _ _ _ _ _]
              tunnel: w2131 -> [_ _ _ _ _ _ _ _ _ _]
              tunnel: w2130 -> [_ _ _ _ _ _ _ _ _ _]
              tunnel: w2129 -> [_ _ _ _ _ _ _ _ _ _]
              tunnel: w2128 -> [w2144 _ _ _ _ _ _ _ _ _]
              tunnel: w2127 -> [_ w2179 _ _ _ _ _ _ _ _]
              tunnel: w2126 -> [_ _ w2219 _ _ _ _ _ _ _]
              tunnel: w2125 -> [_ _ _ w2259 _ _ _ _ _ _]
              tunnel: w2124 -> [_ _ _ _ w2299 _ _ _ _ _]
              tunnel: w2123 -> [_ _ _ _ _ w2339 _ _ _ _]
              tunnel: w2122 -> [_ _ _ _ _ _ w2379 _ _ _]
              tunnel: w2121 -> [_ _ _ _ _ _ _ w2419 _ _]
              tunnel: w2120 -> [_ _ _ _ _ _ _ _ w2459 _]
              tunnel: w2119 -> [_ _ _ _ _ _ _ _ _ w2499]
              frame #0 {
                # "LAB01-1"
